vi "tsdiag_set_filled_byte.vi"(8 "错误输入（无错误）":errorcluster, 9 "pDiagModuleIndex":i32, 10 "AFilledByte":u8, 11 "path":path) -> (0 "错误输出":errorcluster, 2 "Return Type":i32, 3 "path output":path)   [LabVIEW 2014]
doc: "Function Introduction :\nCreate CAN UDS diagnostic service\nCall location :\ninput parameter :\nPDiagModulus Index: Save the int pointer of the UDS module, which is used as a sentence by all diagnostic APIs\nhandle\nAChnIndex: Channel Index\nASupportFDCAN: Does it support FDCAN mode\nAMaxDLC: Maximum data length of canfd frame\nARequestID: request ID for UDS ARequestIDIsStad: whether the request ID is a standard ID AResponseID: response for UDS I AResponseIDIsStad: whether the response ID is a standard ID AFunctionID: UDS function ID AFunctionIDIsStad: whether the function ID is a standard ID\nReturn value :\n==0: Execution successful\nOther values: Query error code"
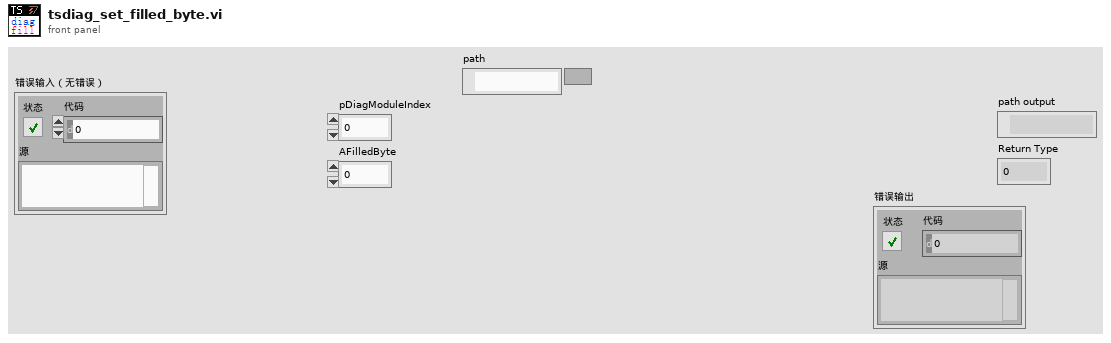
[diagram p1: front panel]
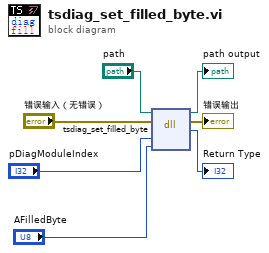
[diagram p0: block diagram]
diagram:
  n1 = dll-call lib="D:/Program Files (x86)/TOSUN/TSMaster/bin/TSMaster.dll" fn="tsdiag_set_filled_byte"(path in="path", error in="错误输入（无错误）", "DiagModuleIndex"="pDiagModuleIndex", "AFilledByte"="AFilledByte") -> (path out=→"path output":path, error out=→"错误输出":errorcluster, "返回类型"=→"Return Type":i32)  [unwired: 3 in]
